vi "AR_Testing.vi"() -> ()   [LabVIEW 2012]
uses:
  BotSpeakSubs/BotspeakSettingsUsed.vi
  SubVIs/LVPresent_Globals.vi
panel:
  in  "Cover":bool
  in  "Analog in channel":u16(ring) items=["A0", "A1", "A2", "A3", "A4", "A5"]
  out "Analog Input":dbl[](graph)
  out "Version":string
  out "Analog":dbl[](array[numeric])
  in  "DIO states":bool[](array[boolean])
  # "Test the Arduino\n\nTry pushing the button or reading a sensor."
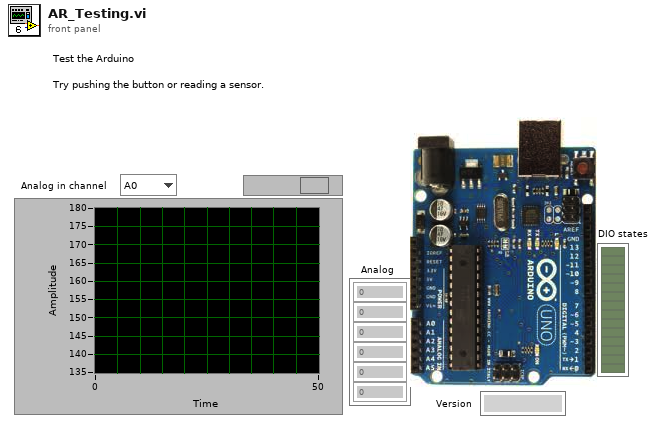
[diagram p1: front panel]
types:
  T1 = typedef "URAPI_Control.ctl" = cluster{"Script":string, "Whiles":u8[], "Ifs":u8[], "Supress Err":bool, "Errors":string}
  T2 = typedef "BotSpeak_Control.ctl" = cluster{"Address":string, "Reply EOF":string, "Hardware":string, "Retries":i8, "Timeout":i32, "Open?":bool}
  T3 = enum8{"Enabled", "Disabled", "Disabled and Grayed Out"}
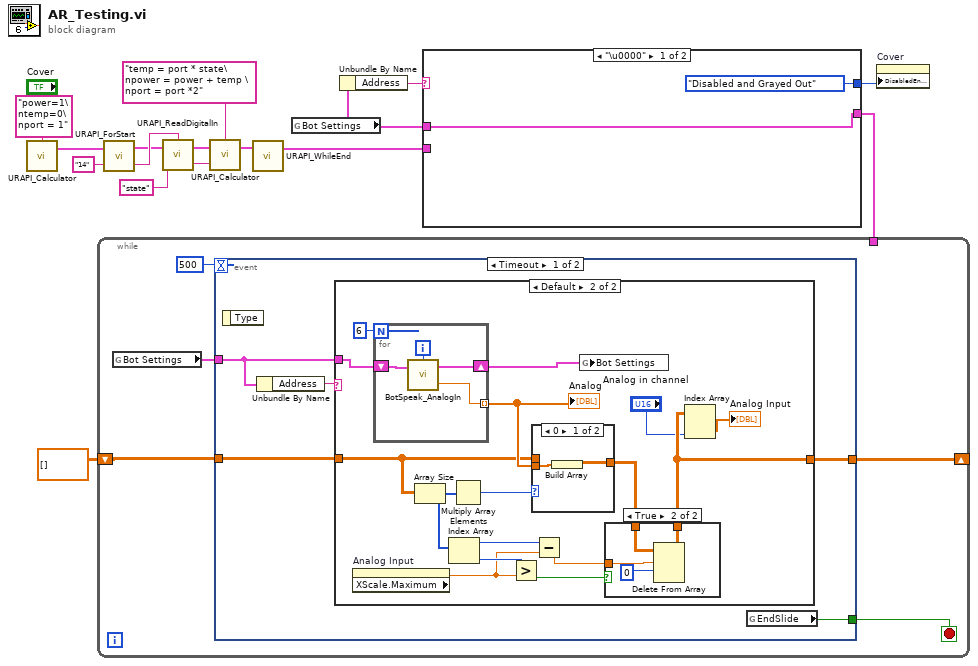
[diagram p0: block diagram]
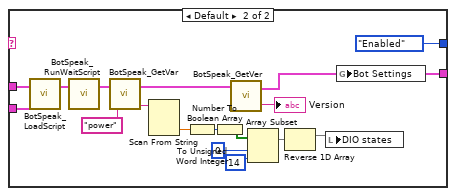
[diagram p2: hidden frame]
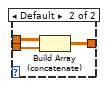
[diagram p5: hidden frame]
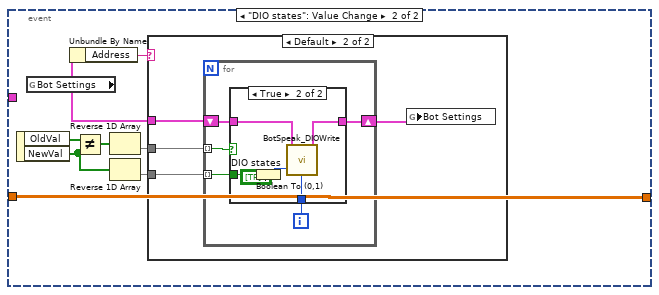
[diagram p6: hidden frame]
diagram:
  n1 = call <userlib>:"URAPI_Calculator.vi"("Formula"="power=1\ntemp=0\nport = 1") -> ("URAPI Script"=w14:T1)  [unwired: 3 in, 1 out]
  n2 = call <userlib>:"URAPI_ForStart.vi"("Iterations"="14", "URAPI Script"=w14) -> ("variable"=w9:string, "URAPI Script Out"=w8:T1)  [unwired: 2 in]
  n3 = call <userlib>:"URAPI_ReadDigitalIn.vi"("Variable In"="state", "URAPI Script"=w8, "Channel"=w9) -> ("Variable Out"=w11:string, "URAPI Script"=w10:T1)  [unwired: 1 in]
  n4 = call <userlib>:"URAPI_Calculator.vi"("X"=w11, "URAPI Script"=w10, "Formula"="temp = port * state\npower = power + temp \nport = port *2") -> ("URAPI Script"=w12:T1)  [unwired: 1 in, 1 out]
  n5 = call <userlib>:"URAPI_WhileEnd.vi"("URAPI Script"=w12) -> ("URAPI Script Out"=w6:T1)  [unwired: 4 in]
  n6 = global read "BotspeakSettingsUsed.vi" "Bot Settings"() -> (w3:T2)
  n7 = Unbundle By Name(w3) -> ("Address"=w2:string)
  n8 = case shown="\"\"" w2 {
    tunnel: w6 -> [_ w22]
    tunnel: [w18 w21] -> w5
    tunnel: w3 -> [w18 w20]
    tunnel: [T3."Disabled and Grayed Out" ("Disabled") T3."Enabled" ("Disabled")] -> w1
    frame "\u0000" {
    }
    frame Default {
      n9 = call <userlib>:"BotSpeak_LoadScript.vi"("URAPI Script"=w22, "Bot Settings"=w20) -> ("Bot Settings"=w25:T2)  [unwired: 1 out]
      n10 = call <userlib>:"BotSpeak_RunWaitScript.vi"("Bot Settings"=w25) -> ("Bot Settings"=w24:T2)  [unwired: 1 in, 1 out]
      n11 = call <userlib>:"BotSpeak_GetVar.vi"("Variable In"="power", "Bot Settings"=w24) -> ("value"=w32:string, "Bot Settings out"=w34:T2)
      n12 = Scan From String(input string=w32) -> (output 1=w26:dbl)  [unwired: 4 in, 3 out]
      n13 = To Unsigned Word Integer(number=w26) -> (unsigned 16bit integer=w31:u16)
      n14 = Number To Boolean Array(number=w31) -> (Boolean array=w29:bool[])
      n15 = call <userlib>:"BotSpeak_GetVer.vi"("Bot Settings"=w34) -> ("version"=→"Version":string, "Bot Settings out"=w21:T2)  [unwired: 1 in]
      n16 = Array Subset(array=w29, index=0, length=14) -> (w30:bool[])
      n17 = Reverse 1D Array(array=w30) -> (reversed array=w33:bool[])
      n18 = local write "DIO states"(w33) -> ()
      n19 = global write "BotspeakSettingsUsed.vi" "Bot Settings"(w21) -> ()
    }
  }
  n20 = while {
    tunnel: w5 -> [_]
    shift-right: [w36] -> _
    shift-left: dbl[][] [] -> [w37]
    stop <- w40 stop-if-true
    n21 = global read "BotspeakSettingsUsed.vi" "Bot Settings"() -> (w38:T2)
    n22 = event shown="[0] Timeout" {
      selector: _ -> [_ _]
      dyn-events: _ -> [_ _]
      timeout: 500 -> [_ _]
      tunnel: [w45 _] -> w40
      tunnel: w38 -> [w44 _]
      tunnel: w37 -> [w42 w76]
      tunnel: [w41 w76] -> w36
      event Timeout {
        n23 = event-data() -> ()  [unwired: 1 in, 1 out]
        n24 = Unbundle By Name(w44) -> ("Address"=w43:string)
        n25 = case shown="Default" w43 {
          tunnel: w44 -> [_ w60]
          tunnel: w42 -> [w46 w54]
          tunnel: [w46 w55] -> w41
          frame "" {
          }
          frame Default {
            n26 = property on="Analog Input" class="WFGraph (strict)"() -> ("XScale.Maximum"=w48:dbl)  [unwired: 2 in, 2 out]
            n27 = for {
              N: 6 -> [_]
              tunnel: [w74] -> w59 mode=indexing
              shift-right: [w72] -> w58
              shift-left: w60 -> [w73]
              i -> [w75]
              n28 = call <userlib>:"BotSpeak_AnalogIn.vi"("Bot Settings"=w73, "A/D Channel"=w75) -> ("voltage"=w74:dbl, "Bot Settings"=w72:T2)  [unwired: 1 in]
            }
            "Analog" <- w59
            n29 = Array Size(array=w54) -> (size(s)=w52:i32[])
            n30 = Index Array(array=w52) -> (element=w49:i32)  [unwired: 1 in]
            n31 = Multiply Array Elements(1:w52) -> (0:w53:i32)
            n32 = Greater?(x=w49, y=w48) -> (0:w51:bool)
            n33 = case shown="0" w53 {
              tunnel: w59 -> [w68 w71]
              tunnel: w54 -> [_ w70]
              tunnel: [w67 w69] -> w57
              frame 0 {
                n34 = Build Array(w68) -> (w67:dbl[][])
              }
              frame Default {
                n35 = Build Array (concatenate)(w70, w71) -> (w69:dbl[][])
              }
            }
            n36 = Subtract(x=w49, y=w48) -> (x-y=w47:dbl)
            n37 = global write "BotspeakSettingsUsed.vi" "Bot Settings"(w58) -> ()
            n38 = case shown="True" w51 {
              tunnel: w57 -> [w62 w66]
              tunnel: [w62 w64] -> w55
              tunnel: w47 -> [_ w63]
              frame False {
              }
              frame True {
                n39 = Delete From Array(array=w66, length=w63, index (row)=0 ("length")) -> (array with subset deleted=w64:dbl[][])  [unwired: 1 in, 1 out]
              }
            }
            n40 = Index Array(array=w55, index (col)="Analog in channel") -> (element=→"Analog Input":dbl[])  [unwired: 1 in]
          }
        }
        n41 = global read "LVPresent_Globals.vi" "EndSlide"() -> (w45:bool)
      }
      event "DIO states": Value Change {
        n42 = event-data() -> ("OldVal"=w80:bool[], "NewVal"=w79:bool[])  [unwired: 1 in]
        n43 = global read "BotspeakSettingsUsed.vi" "Bot Settings"() -> (w83:T2)
        n44 = Unbundle By Name(w83) -> ("Address"=w82:string)
        n45 = Not Equal?(x=w80, y=w79) -> (x != y?=w81:bool[])
        n46 = Reverse 1D Array(array=w81) -> (reversed array=w78:bool[])
        n47 = Reverse 1D Array(array=w79) -> (reversed array=w77:bool[])
        n48 = case shown="Default" w82 {
          tunnel: w83 -> [_ w85]
          tunnel: w78 -> [_ w87]
          tunnel: w77 -> [_ w86]
          frame "" {
          }
          frame Default {
            n49 = for {
              tunnel: w87 -> [w92] mode=indexing
              tunnel: w86 -> [w89] mode=indexing
              shift-right: [w88] -> w84
              shift-left: w85 -> [w90]
              i -> [w91]
              n50 = case shown="True" w92 {
                tunnel: w91 -> [_ w95]
                tunnel: w89 -> [_ w98]
                tunnel: w90 -> [w93 w97]
                tunnel: [w93 w94] -> w88
                frame False {
                }
                frame True {
                  n51 = Boolean To (0,1)(Boolean=w98) -> (0, 1=w96:i16)
                  n52 = call <userlib>:"BotSpeak_DIOWrite.vi"("State"=w96, "Bot Settings"=w97, "DIO Line"=w95) -> ("Bot Settings"=w94:T2)  [unwired: 1 out]
                }
              }
            }
            n53 = global write "BotspeakSettingsUsed.vi" "Bot Settings"(w84) -> ()
          }
        }
      }
    }
  }
  n54 = property on="Cover" class="Bool (strict)"("DisabledEnum"=w1) -> ()  [unwired: 2 in, 2 out]
